vi "Append Section Element.vi"(8 "error in (no error)":errorcluster, 9 "Section":refnum<class "Section.lvclass">, 11 "Configuration in":refnum<class "Configuration.lvclass">) -> (0 "error out":errorcluster, 3 "Configuration out":refnum<class "Configuration.lvclass">)   [LabVIEW 2016, in "Configuration.lvlib" / "Configuration.lvclass"]
doc: "Append section to class private data."
uses:
  Configuration.lvclass
  Section/Section.lvclass
  Configuration.lvclass/Configuration.ctl
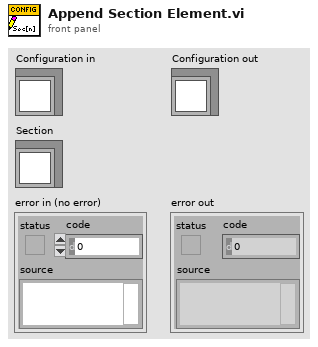
[diagram p1: front panel]
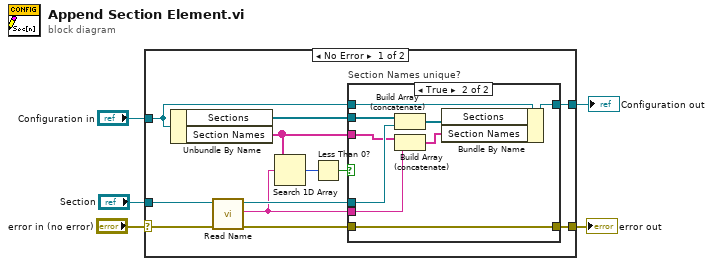
[diagram p0: block diagram]
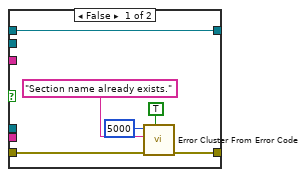
[diagram p2: hidden frame]
diagram:
  n1 = case shown="No Error" "error in (no error)" {
    selector: "error in (no error)" -> [w12 w33]
    tunnel: [w8 w33] -> w4
    tunnel: [w17 w34] -> w2
    tunnel: "Configuration in" -> [w16 w34]
    tunnel: "Section" -> [w14 _]
    frame No Error {
      n2 = Unbundle By Name(w16) -> ("Sections"=w15:refnum<class "Section.lvclass">[], "Section Names"=w11:string[])
      n3 = call "Read Name.vi"("error in (no error)"=w12, "Section in"=w14) -> ("error out"=w9:errorcluster, "Name"=w10:string, "Section out"=w13:refnum<class "Section.lvclass">)  [unwired: 7 in]
      n4 = Search 1D Array(1D array=w11, element=w10) -> (index of element=w7:i32)  [unwired: 1 in]
      n5 = Less Than 0?(x=w7) -> (x < 0?=w6:bool)
      n6 = case "Section Names unique?" shown="True" w6 {
        tunnel: [w23 w32] -> w17
        tunnel: w16 -> [w23 w31]
        tunnel: w15 -> [_ w30]
        tunnel: w13 -> [_ w28]
        tunnel: w11 -> [_ w26]
        tunnel: w10 -> [_ w25]
        tunnel: w9 -> [w22 w24]
        tunnel: [w21 w24] -> w8
        frame False {
          n7 = call <vilib>:"Error Cluster From Error Code.vi"("show call chain? (False)"=TRUE, "error in (no error)"=w22, "error message (\"\")"="Section name already exists." ("error message (\"\")"), "error code (0)"=5000) -> ("error out"=w21:errorcluster)  [unwired: 5 in]
        }
        frame True {
          n8 = Build Array (concatenate)(w30, w28) -> (w29:refnum<class "Section.lvclass">[])
          n9 = Build Array (concatenate)(w26, w25) -> (w27:string[])
          n10 = Bundle By Name(cluster=w31, "Sections"=w29, "Section Names"=w27) -> (w32:refnum<class "Configuration.lvclass">)
        }
      }
    }
    frame Error {
    }
  }
  "error out" <- w4
  "Configuration out" <- w2
